vi "test - Add VI Reference Script.vi"(8 "error in (no error)":errorcluster, 11 "TestCase in":refnum<class "testcase-csmhelper.lvclass">) -> (0 "error out":errorcluster, 3 "TestCase out":refnum<class "testcase-csmhelper.lvclass">)   [LabVIEW 2017, in "testcase-csmhelper.lvclass"]
uses:
  testcase-csmhelper.lvclass
  src/user.lib/_NEVSTOP/Communicable State Machine(CSM)/_csmHelper/CSM-Helper.lvclass/CSM-Helper.ctl
  src/user.lib/_NEVSTOP/Communicable State Machine(CSM)/_csmHelper/Properties/Read VI Ref.vi
  src/user.lib/_NEVSTOP/Communicable State Machine(CSM)/_csmHelper/Properties/Read States.vi
  src/user.lib/_NEVSTOP/Communicable State Machine(CSM)/_csmHelper/API/Undo.vi
  src/user.lib/_NEVSTOP/Communicable State Machine(CSM)/_csmHelper/API/Remove State Frame.vi
  src/user.lib/_NEVSTOP/Communicable State Machine(CSM)/_csmHelper/API/Open Block Diagram.vi
  src/user.lib/_NEVSTOP/Communicable State Machine(CSM)/_csmHelper/API/Add VI Reference Case.vi
  src/user.lib/_NEVSTOP/Communicable State Machine(CSM)/_csmHelper/API/Stop Undo.vi
  src/user.lib/_NEVSTOP/Communicable State Machine(CSM)/_csmHelper/API/Start Undo.vi
  src/user.lib/_NEVSTOP/Communicable State Machine(CSM)/_csmHelper/API/Destroy.vi
  src/user.lib/_NEVSTOP/Communicable State Machine(CSM)/_csmHelper/API/Create From VI Reference.vi
  <vilib>/addons/_JKI Toolkits/VI Tester/TestCase.llb/TestCase.lvclass
  src/user.lib/_NEVSTOP/Communicable State Machine(CSM)/_csmHelper/CSM-Helper.lvclass
  C:/Program Files (x86)/National Instruments/LabVIEW 2017/vi.lib/addons/_JKI Toolkits/VI Tester/TestCase.llb/TestCase.lvclass
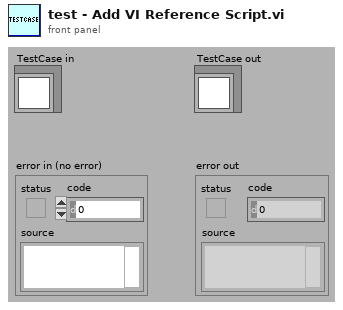
[diagram p1: front panel]
types:
  T1 = enum32{"Bad", "Idle", "Run top level", "Running"}
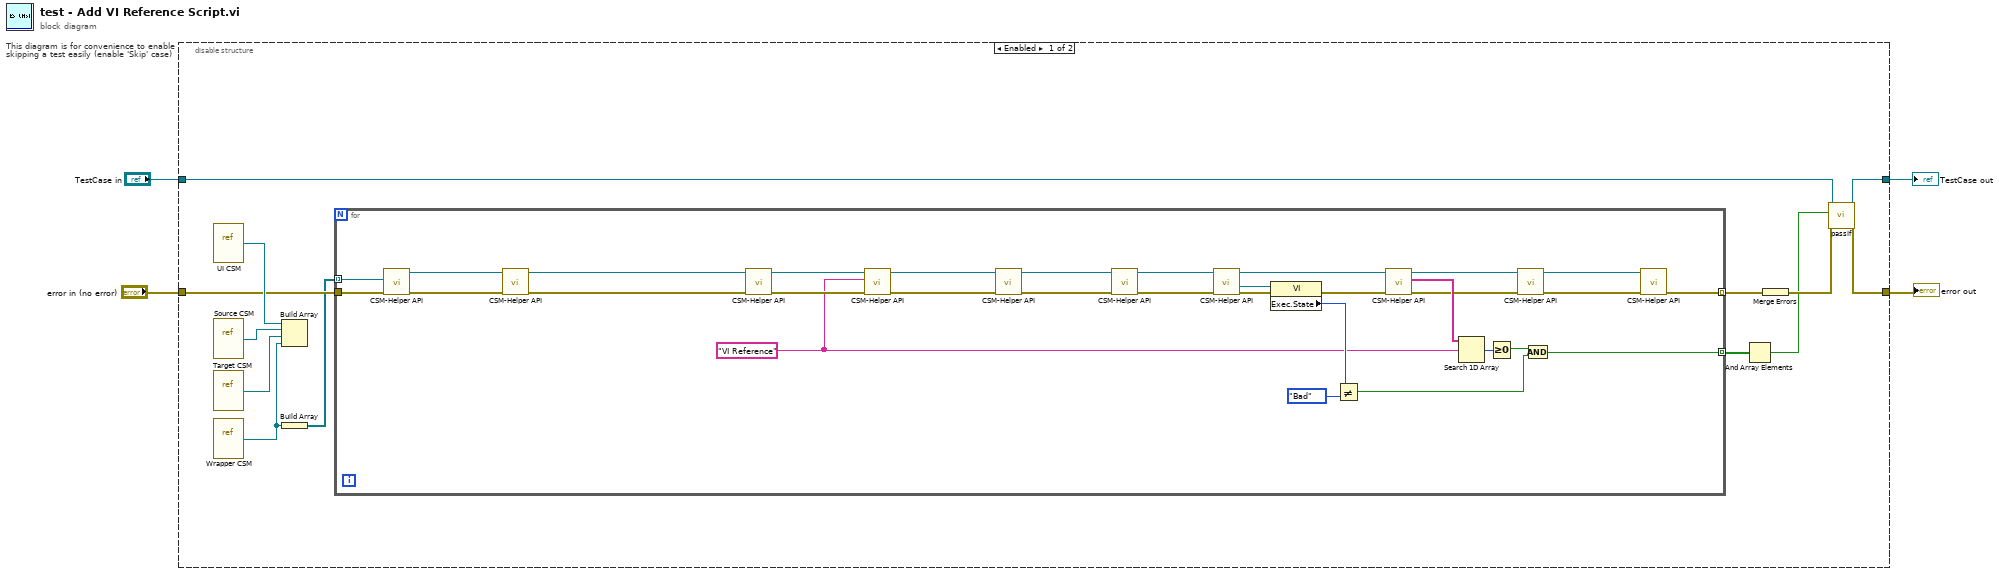
[diagram p0: block diagram]
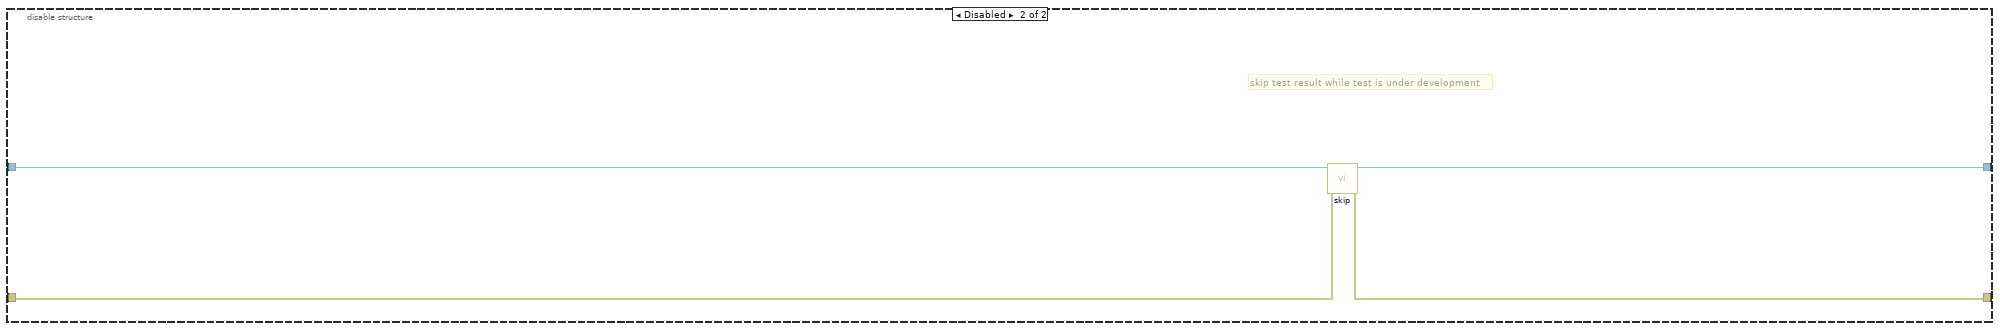
[diagram p2: hidden frame]
diagram:
  n1 = disable-structure "This diagram is for convenience to enable skipping a test easily (enable 'Skip' case)" shown="Enabled" {
    disable-tunnel: "TestCase in" -> [w17 w52]
    disable-tunnel: [w16 w50] -> w1
    disable-tunnel: [w15 w51] -> w3
    disable-tunnel: "error in (no error)" -> [w12 w49]
    frame Enabled {
      n2 = vi-ref "UI CSM.vi"() -> (w14:refnum<vi>)
      n3 = vi-ref "Source CSM.vi"() -> (w8:refnum<vi>)
      n4 = vi-ref "Target CSM.vi"() -> (w7:refnum<vi>)
      n5 = vi-ref "Wrapper CSM.vi"() -> (w6:refnum<vi>)
      n6 = Build Array(w14, w8, w7, w6) -> ()  [unwired: 1 out]
      n7 = Build Array(w6) -> (w5:refnum<vi>[])
      n8 = for {
        tunnel: w5 -> [w48] mode=indexing
        tunnel: [w47] -> w13 mode=indexing
        tunnel: w12 -> [w46]
        tunnel: [w45] -> w11 mode=indexing
        w18 = "VI Reference" ("element")
        n9 = call-poly "CSM-Helper API.vi"("error in (no error)"=w46, "VI"=w48) -> ("error out"=w22:errorcluster, "CSM-Helper.lvclass"=w21:refnum<class "CSM-Helper.lvclass">)  [unwired: 8 in]
        n10 = call-poly "CSM-Helper API.vi"("error in (no error)"=w22, "CSM-Helper in"=w21) -> ("error out"=w20:errorcluster, "CSM-Helper out"=w19:refnum<class "CSM-Helper.lvclass">)  [unwired: 8 in]
        n11 = call-poly "CSM-Helper API.vi"("error in (no error)"=w20, "CSM-Helper in"=w19) -> ("error out"=w23:errorcluster, "CSM-Helper out"=w24:refnum<class "CSM-Helper.lvclass">)  [unwired: 8 in]
        n12 = call-poly "CSM-Helper API.vi"("error in (no error)"=w23, "element"=w18, "CSM-Helper in"=w24) -> ("error out"=w26:errorcluster, "CSM-Helper out"=w25:refnum<class "CSM-Helper.lvclass">)  [unwired: 7 in]
        n13 = call-poly "CSM-Helper API.vi"("error in (no error)"=w26, "CSM-Helper in"=w25) -> ("error out"=w41:errorcluster, "CSM-Helper out"=w42:refnum<class "CSM-Helper.lvclass">)  [unwired: 8 in]
        n14 = call-poly "CSM-Helper API.vi"("error in (no error)"=w41, "CSM-Helper in"=w42) -> ("error out"=w40:errorcluster, "CSM-Helper out"=w39:refnum<class "CSM-Helper.lvclass">)  [unwired: 8 in]
        n15 = call-poly "CSM-Helper API.vi"("error in (no error)"=w40, "CSM-Helper in"=w39) -> ("error out"=w38:errorcluster, "VI"=w37:refnum<vi>, "CSM-Helper out"=w30:refnum<class "CSM-Helper.lvclass">)  [unwired: 7 in]
        n16 = property class="VI"(reference=w37, error in=w38) -> (error out=w31:errorcluster, "Exec.State"=w36:T1)  [unwired: 1 out]
        n17 = Not Equal?(x=w36, y=T1."Bad") -> (x != y?=w34:bool)
        n18 = call-poly "CSM-Helper API.vi"("error in (no error)"=w31, "CSM-Helper in"=w30) -> ("error out"=w27:errorcluster, "Value"=w32:string[], "CSM-Helper out"=w28:refnum<class "CSM-Helper.lvclass">)  [unwired: 7 in]
        n19 = Search 1D Array(1D array=w32, element=w18) -> (index of element=w33:i32)  [unwired: 1 in]
        n20 = Greater Or Equal To 0?(x=w33) -> (x >= 0?=w29:bool)
        n21 = call-poly "CSM-Helper API.vi"("error in (no error)"=w27, "CSM-Helper in"=w28) -> ("error out"=w43:errorcluster, "CSM-Helper out"=w44:refnum<class "CSM-Helper.lvclass">)  [unwired: 8 in]
        n22 = And(x=w29, y=w34) -> (x .and. y?=w47:bool)
        n23 = call-poly "CSM-Helper API.vi"("error in (no error)"=w43, "CSM-Helper in"=w44) -> ("error out"=w45:errorcluster)  [unwired: 8 in, 1 out]
      }
      n24 = And Array Elements(Boolean array=w13) -> (logical AND=w9:bool)
      n25 = Merge Errors(w11) -> (w10:errorcluster)
      n26 = call-dynamic "passIf.vi"("error in (no error)"=w10, "pass"=w9, "TestCase in"=w17) -> ("error out"=w15:errorcluster, "TestCase out"=w16:refnum<class "testcase-csmhelper.lvclass">)  [unwired: 7 in]
    }
    frame Disabled {
      # "skip test result while test is under development"
      n27 = call <vilib>:"skip.vi"("error in (no error)"=w49, "TestCase in"=w52) -> ("error out"=w51:errorcluster, "TestCase out"=w50:refnum<class "testcase-csmhelper.lvclass">)  [unwired: 8 in]
    }
  }
  "error out" <- w3
  "TestCase out" <- w1
